vi "Read Encoder Speed RPM.vi"(8 "error in (no error)":errorcluster, 10 "channel number":u8, 11 "VISA resource name":refnum<visa-resource-name>) -> (0 "error out":errorcluster, 2 "Encoder Speed (RPM)":i32, 3 "VISA resource name out":refnum<visa-resource-name>)   [LabVIEW 2012, in "Roboteq.lvlib"]
uses:
  Roboteq.lvlib
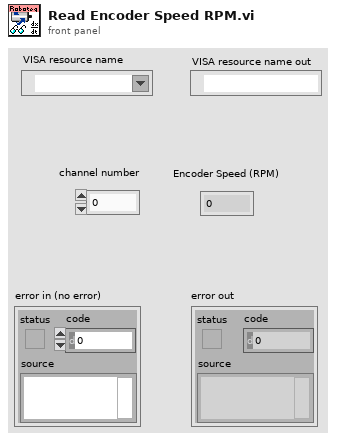
[diagram p1: front panel]
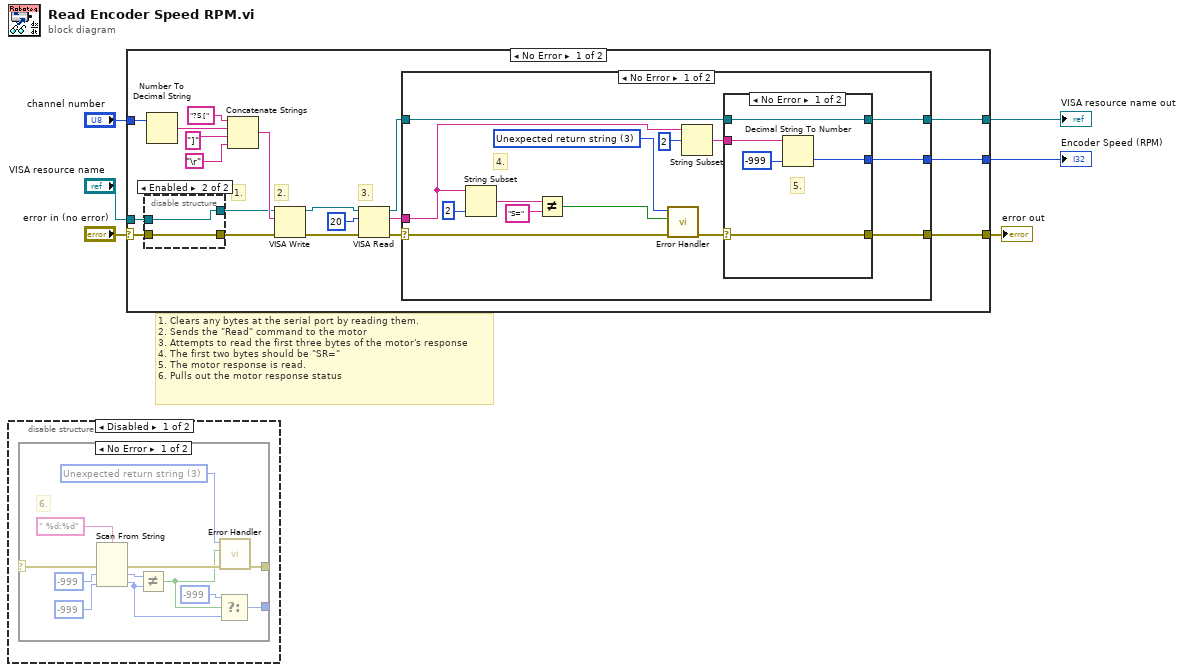
[diagram p0: block diagram]
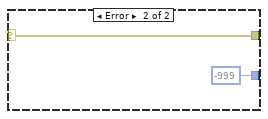
[diagram p2: hidden frame]
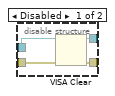
[diagram p4: hidden frame]
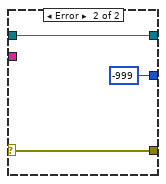
[diagram p5: hidden frame]
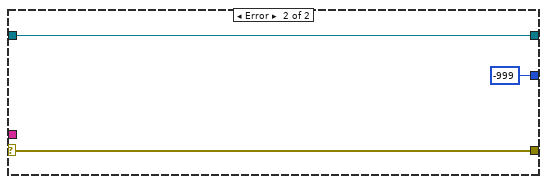
[diagram p6: hidden frame]
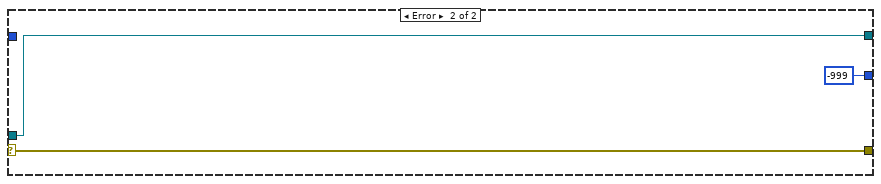
[diagram p7: hidden frame]
diagram:
  # "1. Clears any bytes at the serial port by reading them.\n2. Sends the \"Read\" command to the motor\n3. Attempts to read the first three bytes of the motor's response\n4. The first two bytes should be \"SR=\"\n5. The motor response is read.\n6. Pulls out the motor response status"
  n1 = disable-structure shown="Disabled" {
    frame Disabled {
      n2 = case shown="No Error" {
        selector: _ -> [w16 w19]
        tunnel: [w14 w19] -> _
        tunnel: [w11 -999 ("main battery\nvoltage (V)")] -> _
        frame No Error {
          w12 = u16 3 items=["Scan timeout"=1, "Invalid motor checksum"=2, "Unexpected return string"=3, "Invalid address range"=4] ("Error type")
          # "6."
          n3 = Scan From String(format string=" %d:%d", error in=w16, default 1=-999 ("default value 1"), default 2=-999 ("default value 1")) -> (error out=w13:errorcluster, output 1=w10:i32, output 2=w7:i32)  [unwired: 2 in, 2 out]
          n4 = Not Equal?(x=w10, y=w7) -> (x != y?=w8:bool)
          n5 = Select(t=-999 ("default value 1"), s=w8, f=w7) -> (s? t:f=w11:i32)
          n6 = call "Error Handler.vi"("error in (no error)"=w13, "Error? (no error)"=w8, "Error type"=w12) -> ("error out"=w14:errorcluster)  [unwired: 8 in]
        }
        frame Error {
        }
      }
    }
    frame Enabled {
    }
  }
  n7 = case shown="No Error" "error in (no error)" {
    selector: "error in (no error)" -> [w23 w73]
    tunnel: [w31 w73] -> w5
    tunnel: [w32 -999 ("main battery\nvoltage (V)")] -> w2
    tunnel: "VISA resource name" -> [w24 w71]
    tunnel: [w30 w71] -> w3
    tunnel: "channel number" -> [w26 _]
    frame No Error {
      # "3."
      # "2."
      # "1."
      n8 = disable-structure shown="Enabled" {
        disable-tunnel: w24 -> [w43 w44]
        disable-tunnel: w23 -> [w42 w45]
        disable-tunnel: [w41 w44] -> w22
        disable-tunnel: [w40 w45] -> w21
        frame Disabled {
          n9 = VISA Clear(VISA resource name=w43, error in (no error)=w42) -> (VISA resource name out=w41:refnum<visa-resource-name>, error out=w40:errorcluster)
        }
        frame Enabled {
        }
      }
      n10 = Number To Decimal String(number=w26) -> (decimal integer string=w25:string)  [unwired: 1 in]
      n11 = Concatenate Strings("?S [" ("string"), w25, "]" ("string"), "\r") -> (w39:string)
      n12 = VISA Write(VISA resource name=w22, write buffer=w39, error in (no error)=w21) -> (VISA resource name out=w37:refnum<visa-resource-name>, error out=w36:errorcluster)  [unwired: 1 out]
      n13 = VISA Read(VISA resource name=w37, byte count=u32 20, error in (no error)=w36) -> (VISA resource name out=w34:refnum<visa-resource-name>, read buffer=w33:string, error out=w35:errorcluster)  [unwired: 1 out]
      n14 = case shown="No Error" w35 {
        selector: w35 -> [w55 w70]
        tunnel: w33 -> [w48 _]
        tunnel: [w57 w70] -> w31
        tunnel: w34 -> [w59 w69]
        tunnel: [w58 w69] -> w30
        tunnel: [w51 -999 ("main battery\nvoltage (V)")] -> w32
        frame No Error {
          w52 = u16 3 items=["Scan timeout"=1, "Invalid motor checksum"=2, "Unexpected return string"=3, "Invalid address range"=4] ("Error type")
          # "4."
          n15 = String Subset(string=w48, length (rest)=2 ("length (rest)")) -> (substring=w47:string)  [unwired: 1 in]
          n16 = Not Equal?(x=w47, y="S=" ("string")) -> (x != y?=w54:bool)
          n17 = call "Error Handler.vi"("error in (no error)"=w55, "Error? (no error)"=w54, "Error type"=w52) -> ("error out"=w56:errorcluster)  [unwired: 8 in]
          n18 = String Subset(string=w48, offset (0)=2 ("length (rest)")) -> (substring=w46:string)  [unwired: 1 in]
          n19 = case shown="No Error" w56 {
            selector: w56 -> [w60 w66]
            tunnel: w59 -> [w64 w67]
            tunnel: [w64 w67] -> w58
            tunnel: [w60 w66] -> w57
            tunnel: [w61 -999 ("main battery\nvoltage (V)")] -> w51
            tunnel: w46 -> [w63 _]
            frame No Error {
              # "5."
              n20 = Decimal String To Number(string=w63, default (0L)=-999 ("default (0 I32)")) -> (number=w61:i32)  [unwired: 1 in, 1 out]
            }
            frame Error {
            }
          }
        }
        frame Error {
        }
      }
    }
    frame Error {
    }
  }
  "VISA resource name out" <- w3
  "error out" <- w5
  "Encoder Speed (RPM)" <- w2
